vi "main.vi"() -> ()   [LabVIEW 2020]
uses:
  subvi/status/status of power_supply3.vi
  subvi/status/status of power_supply4.vi
  subvi/status/status of power_supply2.vi
  subvi/status/status of power_supply1.vi
  subvi/status/status of pump.vi
  subvi/status/status of relay.vi
  subvi/status/status of robot.vi
  subvi/status/status of worker2.vi
  subvi/status/status of worker4.vi
  subvi/status/status of worker3.vi
  subvi/status/status of worker1.vi
  subvi/status/item name.vi
  subvi/status/public_device_list.vi
  subvi/status/item name2.vi
  subvi/status/robot pause.vi
  subvi/status/stop software.vi
  subvi/status/emergency stop.vi
  subvi/status/filter_vial_No.vi
  subvi/status/skip_latter.vi
  subvi/status/skip_status.vi
  subvi/status/pause1.vi
  subvi/status/pause3.vi
  subvi/status/pause2.vi
  subvi/status/pause4.vi
  subvi/status/time1.vi
  subvi/status/time2.vi
  subvi/status/time3.vi
  subvi/status/time4.vi
  subvi/status/experiment_No.vi
  <vilib>/NI/Modbus Library/API/Wrapper/Create Serial Master.vi
  subvi/robot/subvi/Robot-HL/small_scara_interface/small_scara_interface.lvlib
  <vilib>/NI/Modbus Library/API/Wrapper/API Main.lvlib
panel:
  in  "robot pause":bool
  in  "stop software":bool
  in  "emergency stop":bool
  in  "Main interface":T1(tab)
  in  "release occupy":bool
  in  "pump load":bool
  in  "power_supply2 load":bool
  in  "motor load":bool
  in  "power_supply1 load":bool
  in  "robot load":bool
  in  "power_supply2":refnum<visa-resource-name>
  in  "power_supply":refnum<visa-resource-name>
  out "robot_busy/ready":bool
  out "pump_busy/ready":bool
  out "worker1_busy/ready":bool
  out "worker2_busy/ready":bool
  out "worker3_busy/ready":bool
  out "worker4_busy/ready":bool
  in  "start":bool
  in  "user.xls path":path=path "C:/Users/Mogroup-3/Desktop/AutoChem_test/user.xls"
  in  "Python version":string="3.11"
  out "power_supply4_busy/ready":bool
  out "power_supply1_busy/ready":bool
  out "power_supply3_busy/ready":bool
  out "power_supply2_busy/ready":bool
  out "filter_vial_No":i32
  out "relay_busy/ready":bool
  in  "pump":refnum<visa-resource-name>
  in  "motor":refnum<visa-resource-name>
  in  "filter_vial_No initial":i32
  in  "pause4":bool
  in  "pause2":bool
  in  "pause3":bool
  in  "pause1":bool
  in  "Refresh":bool
  in  "device log":i32(listbox)
  in  "experiment information":i32(listbox)
  out "start time 1":timestamp
  out "during time 1/s":dbl
  out "start time 2":timestamp
  out "during time 2/s":dbl
  out "start time 3":timestamp
  out "start time 4":timestamp
  out "during time 3/s":dbl
  out "during time 4/s":dbl
  in  "pump test":bool
  in  "channel":string
  in  "volume":dbl
  in  "rate":dbl
  in  "wait_time":dbl
  in  "robot run":bool
  in  "robot axis read":bool
  out "resulting string":string
  in  "distance":sgl
  in  "x":sgl
  in  "y":sgl
  in  "z":sgl
  in  "r":sgl
  in  "speed":sgl
  in  "rough":sgl
  in  "motor test":bool
  in  "motor ID":u8
  in  "motor commamd":string
  in  "rotate rate":u16
  in  "power_supply test":bool
  in  "Channel (1: Channel 1)":i32(ring)=1 items=["Channel 1"=1, "Channel 2"=2]
  in  "command":string
  in  "Enable Output (T: Enable)":bool=TRUE
  in  "Channel (1: Channel 1) 2":i32(ring)=1 items=["Channel 1"=1, "Channel 2"=2]
  in  "command 2":string
  in  "power_supply test 2":bool
  in  "Enable Output (T: Enable) 2":bool=TRUE
  # "Connection COM ports table"
  # "power_supply_busy/ready"
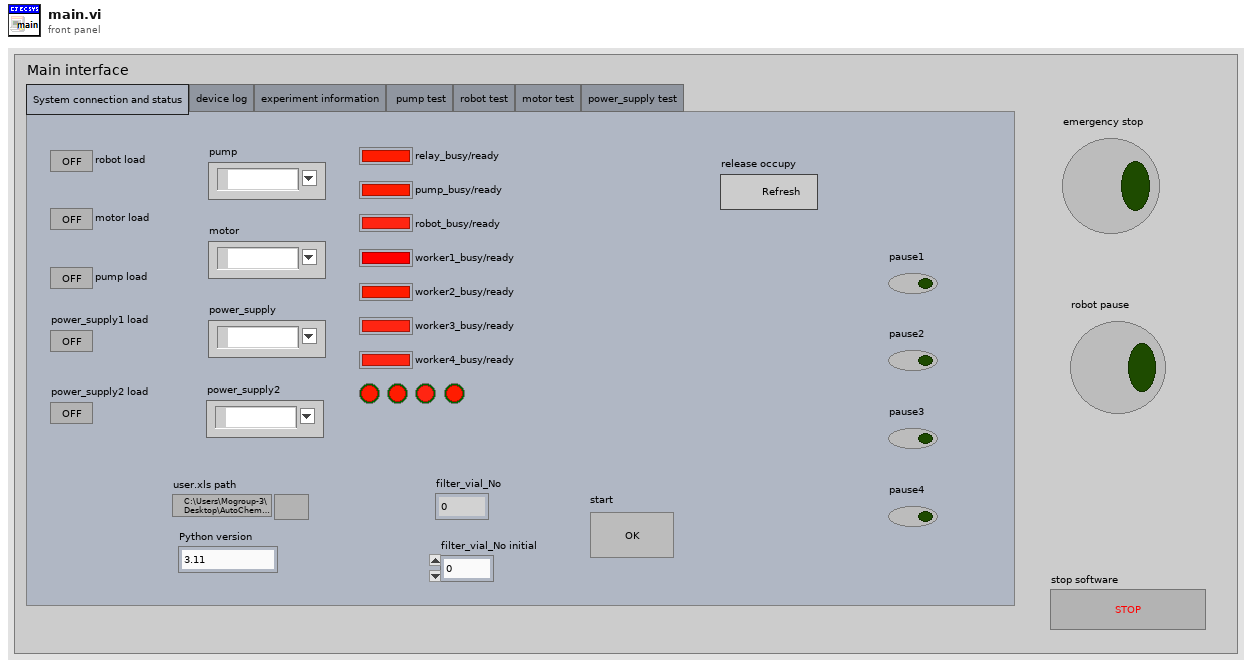
[diagram p1: front panel]
types:
  T1 = enum32{"System connection and status", "device log", "experiment information", " pump test", "robot test", "motor test", "power_supply test"}
  T2 = cluster{"start time 1":timestamp, "during time 1/s":dbl}
  T3 = cluster{"start time 2":timestamp, "during time 2/s":dbl}
  T4 = cluster{"start time 3":timestamp, "during time 3/s":dbl}
  T5 = cluster{"start time 4":timestamp, "during time 4/s":dbl}
  T6 = cluster{"x":sgl, "y":sgl, "z":sgl, "angle1":sgl, "angle2":sgl, "rotation":sgl}
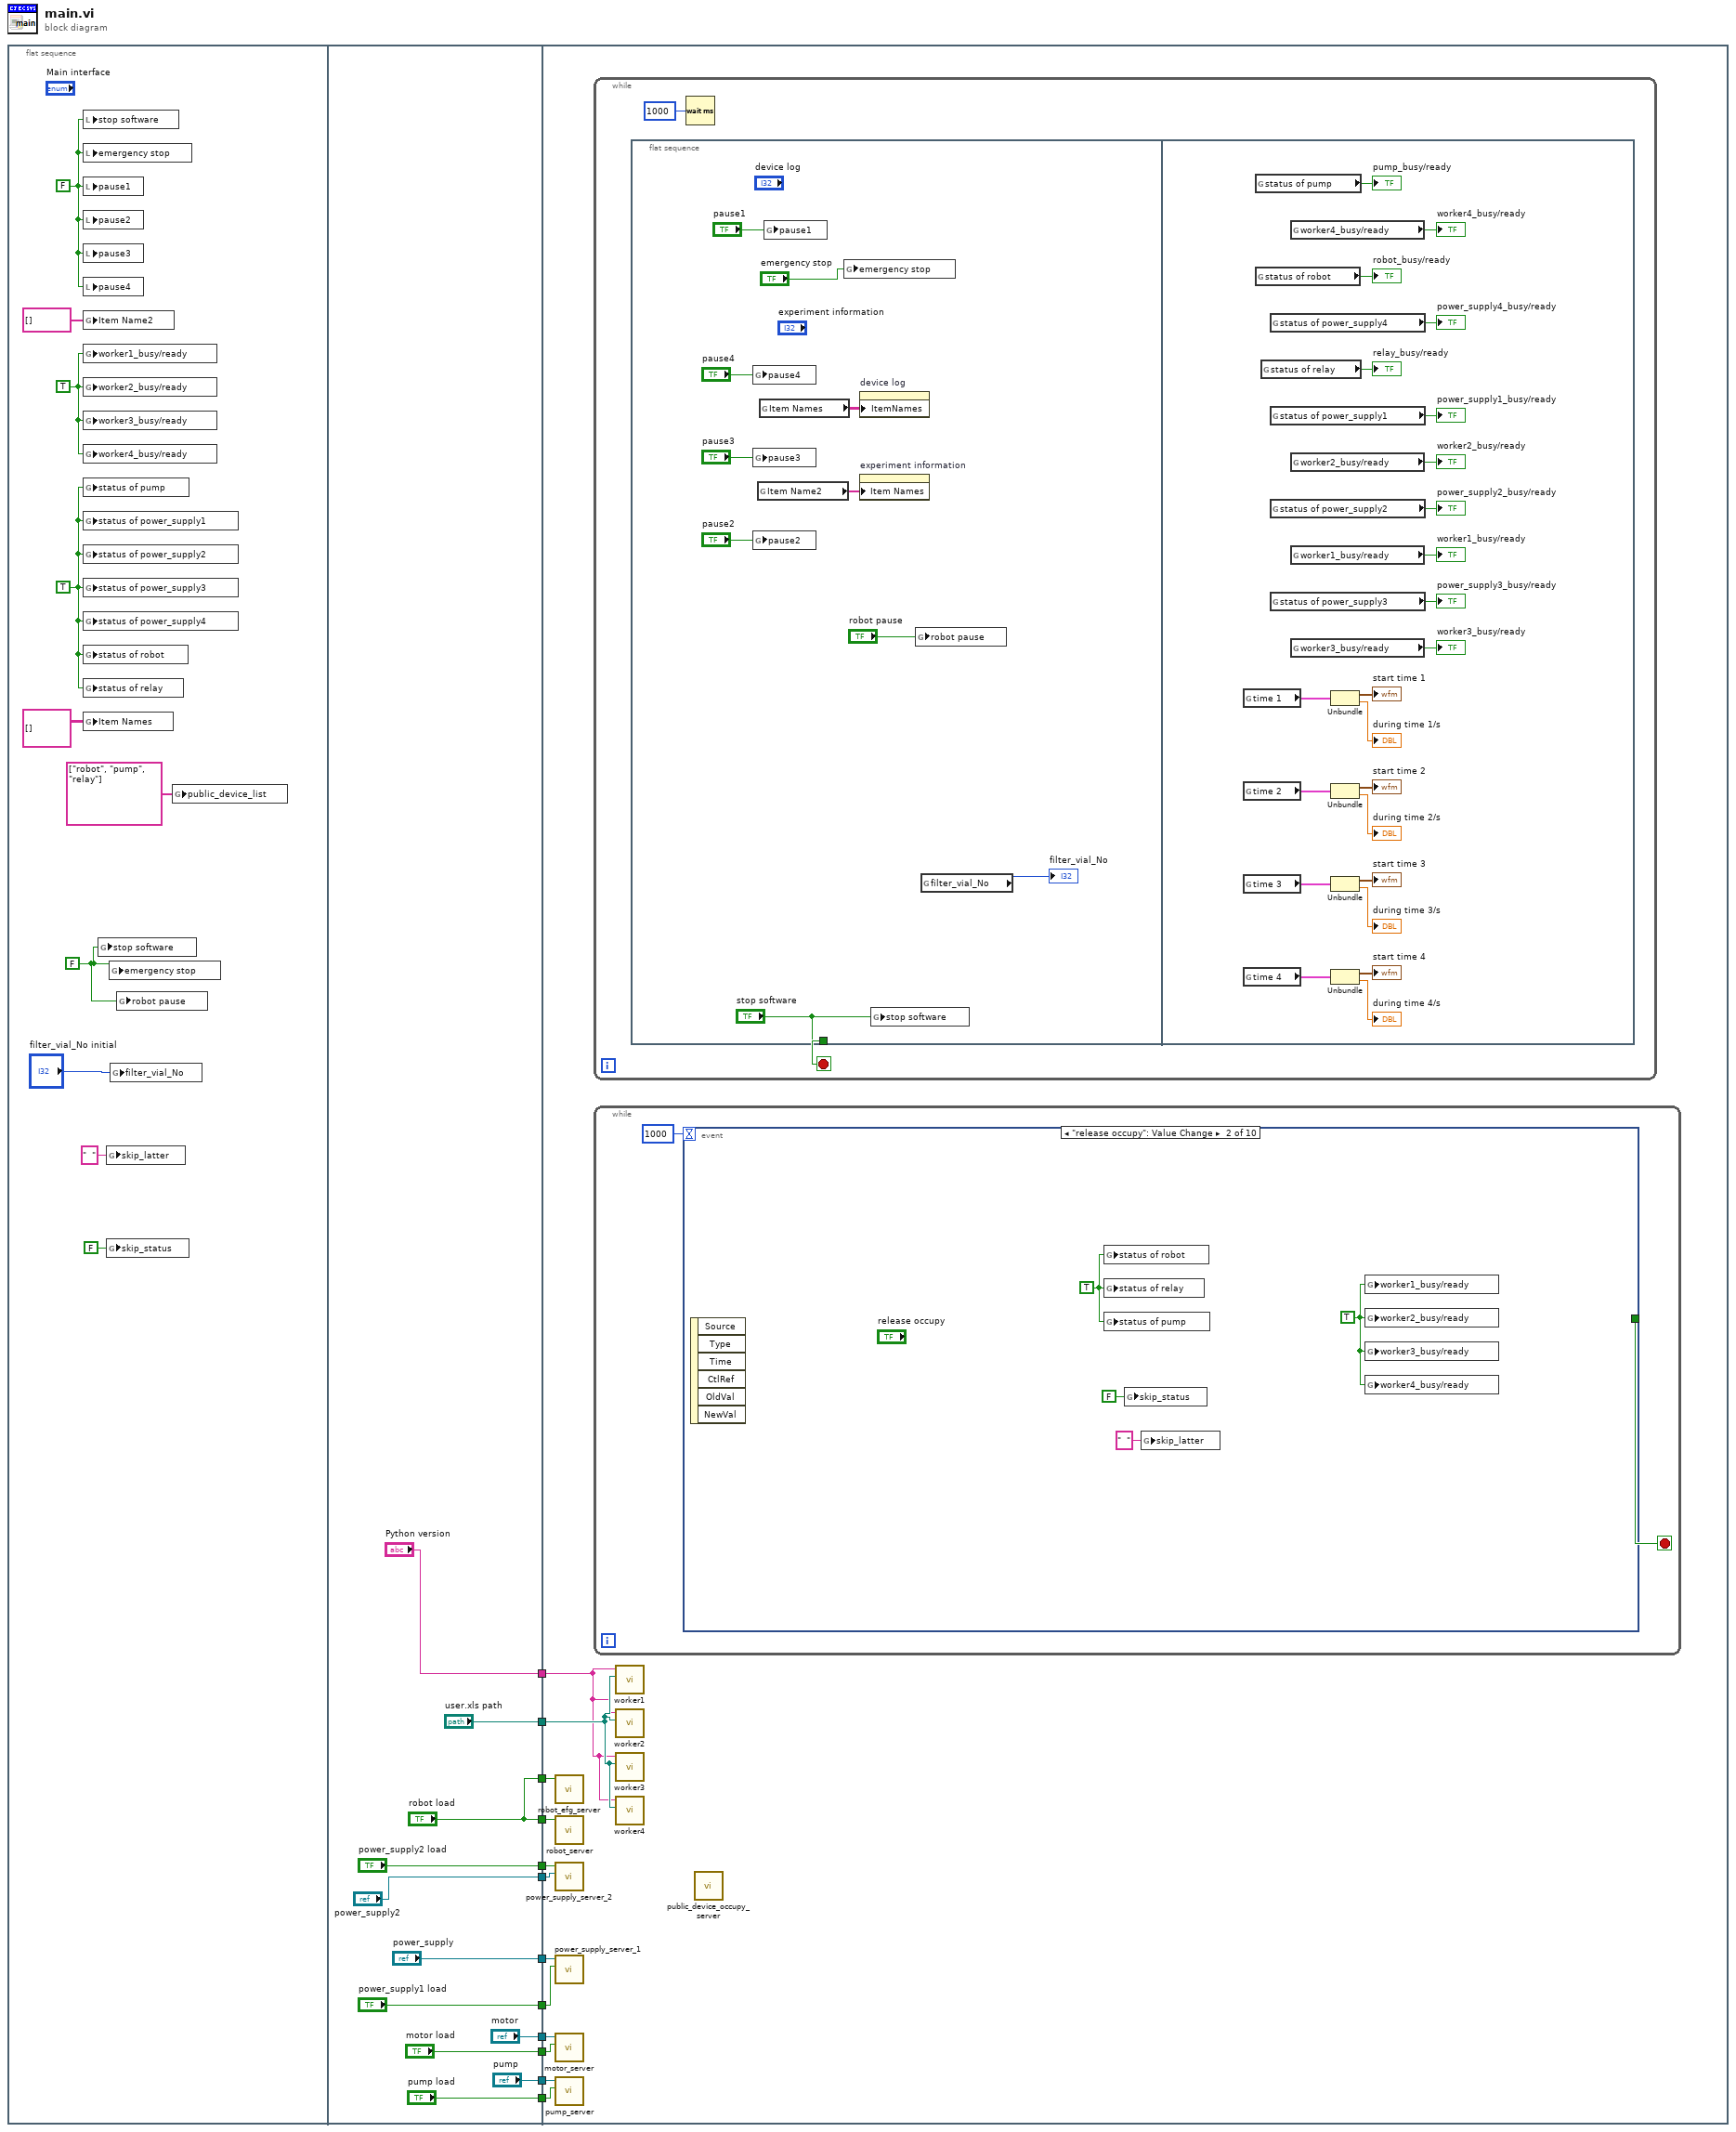
[diagram p0: block diagram]
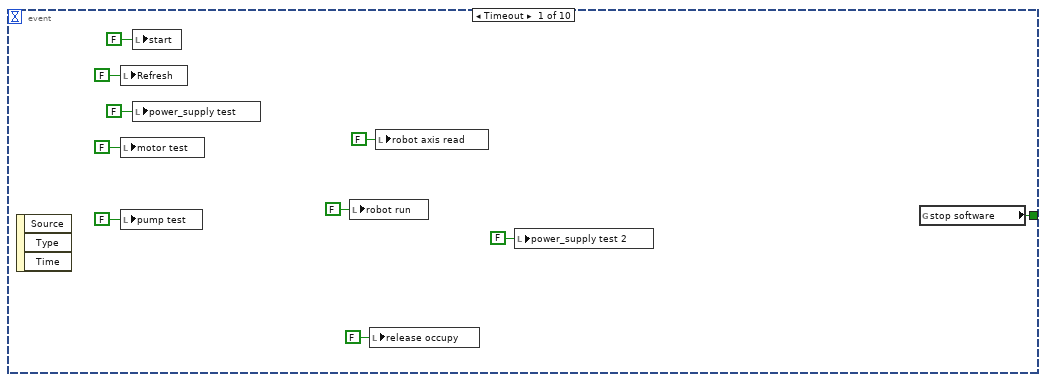
[diagram p2: hidden frame]
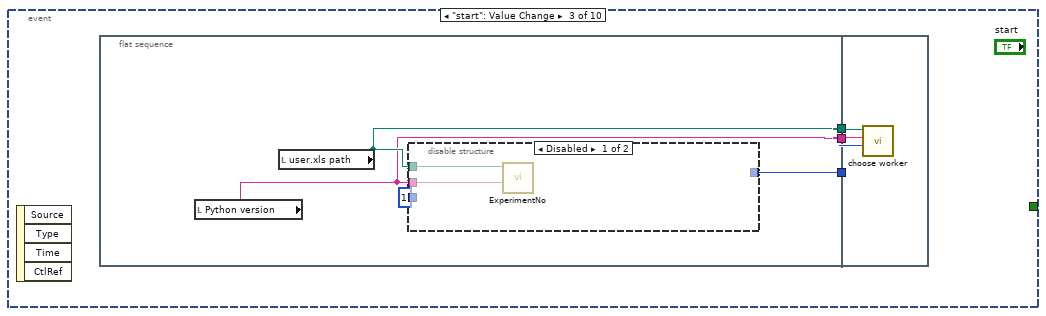
[diagram p3: hidden frame]
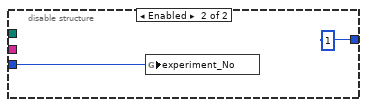
[diagram p4: hidden frame]
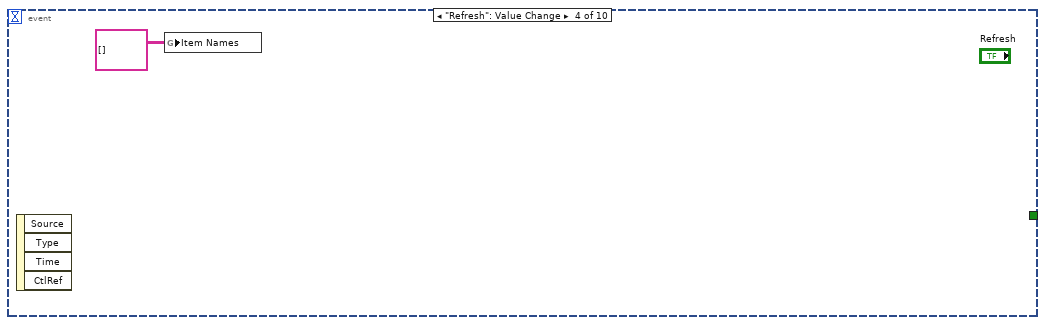
[diagram p5: hidden frame]
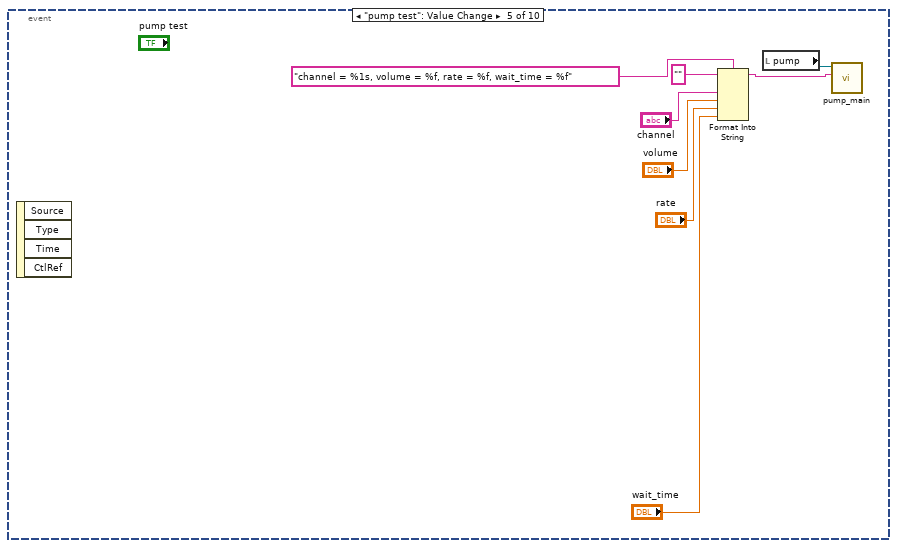
[diagram p6: hidden frame]
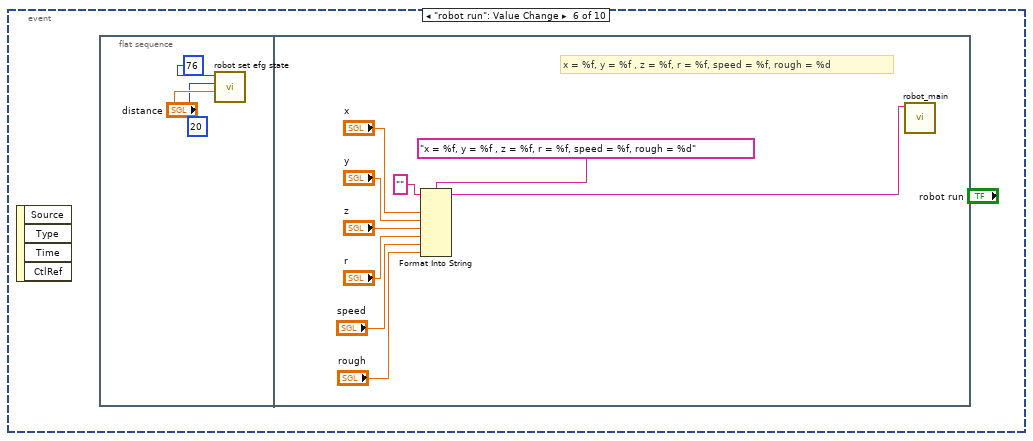
[diagram p7: hidden frame]
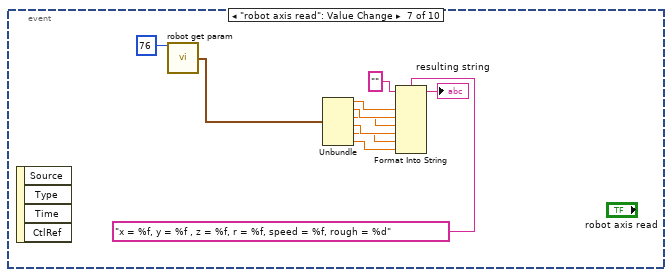
[diagram p8: hidden frame]
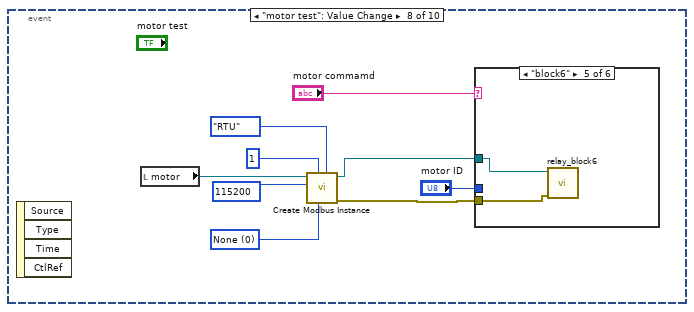
[diagram p9: hidden frame]
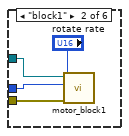
[diagram p11: hidden frame]
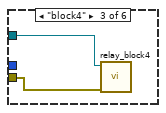
[diagram p12: hidden frame]
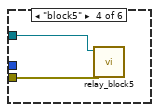
[diagram p13: hidden frame]
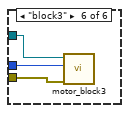
[diagram p14: hidden frame]
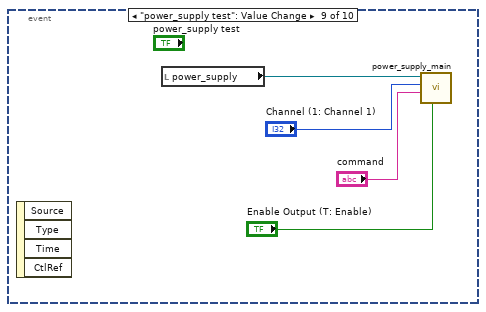
[diagram p15: hidden frame]
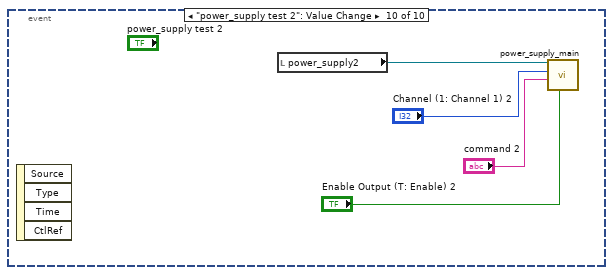
[diagram p16: hidden frame]
diagram:
  n1 = flat-sequence {
    tunnel: ["power_supply"] -> w12
    tunnel: ["motor"] -> w11
    tunnel: ["pump"] -> w10
    tunnel: ["robot load"] -> w9
    tunnel: ["power_supply1 load"] -> w8
    tunnel: ["motor load"] -> w7
    tunnel: ["pump load"] -> w6
    tunnel: ["power_supply2 load"] -> w5
    tunnel: ["power_supply2"] -> w4
    tunnel: ["user.xls path"] -> w3
    tunnel: ["Python version"] -> w2
    tunnel: ["robot load"] -> w1
    tunnel: w12 -> [w45]
    tunnel: w11 -> [w44]
    tunnel: w10 -> [w43]
    tunnel: w9 -> [w42]
    tunnel: w8 -> [w41]
    tunnel: w7 -> [w40]
    tunnel: w6 -> [w39]
    tunnel: w5 -> [w37]
    tunnel: w4 -> [w36]
    tunnel: w3 -> [w35]
    tunnel: w2 -> [w34]
    tunnel: w1 -> [w38]
    frame #0 {
      w15 = FALSE ("emergency stop")
      w21 = TRUE ("worker1_busy/ready")
      w19 = TRUE ("status of pump")
      w18 = FALSE ("stop software")
      n2 = local write "stop software"(w18) -> ()
      n3 = local write "emergency stop"(w18) -> ()
      n4 = local write "pause1"(w18) -> ()
      n5 = local write "pause2"(w18) -> ()
      n6 = local write "pause3"(w18) -> ()
      n7 = local write "pause4"(w18) -> ()
      n8 = global write "item name2.vi" "Item Name2"(string[] [] ("Item Name2")) -> ()
      n9 = global write "status of worker1.vi" "worker1_busy/ready"(w21) -> ()
      n10 = global write "status of worker2.vi" "worker2_busy/ready"(w21) -> ()
      n11 = global write "status of worker3.vi" "worker3_busy/ready"(w21) -> ()
      n12 = global write "status of worker4.vi" "worker4_busy/ready"(w21) -> ()
      n13 = global write "status of pump.vi" "status of pump"(w19) -> ()
      n14 = global write "status of power_supply1.vi" "status of power_supply1"(w19) -> ()
      n15 = global write "status of power_supply2.vi" "status of power_supply2"(w19) -> ()
      n16 = global write "status of power_supply3.vi" "status of power_supply3"(w19) -> ()
      n17 = global write "status of power_supply4.vi" "status of power_supply4"(w19) -> ()
      n18 = global write "status of robot.vi" "status of robot"(w19) -> ()
      n19 = global write "status of relay.vi" "status of relay"(w19) -> ()
      n20 = global write "item name.vi" "Item Names"(string[][] [] ("Item Names")) -> ()
      n21 = global write "stop software.vi" "stop software"(w15) -> ()
      n22 = global write "skip_latter.vi" "skip_latter"("  " ("skip_latter")) -> ()
      n23 = global write "skip_status.vi" "skip_status"(FALSE ("skip_status")) -> ()
      n24 = global write "emergency stop.vi" "emergency stop"(w15) -> ()
      n25 = global write "filter_vial_No.vi" "filter_vial_No"("filter_vial_No initial") -> ()
      n26 = global write "robot pause.vi" "robot pause"(w15) -> ()
      n27 = global write "public_device_list.vi" "public_device_list"(string[] ["robot", "pump", "relay"] ("Array")) -> ()
    }
    frame #1 {
    }
    frame #2 {
      n28 = call "robot_efg_server.vi"("efg load"=w38) -> ()  [unwired: 11 in]
      n29 = call "robot_server.vi"("robot load"=w42) -> ()  [unwired: 11 in]
      n30 = call "power_supply_server_2.vi"("power_supply 3&4"=w36, "power_supply2 load"=w37) -> ()  [unwired: 10 in]
      n31 = call "power_supply_server_1.vi"("power_supply1 load"=w41, "power_supply 1&2"=w45) -> ()  [unwired: 10 in]
      n32 = call "motor_server.vi"("motor load"=w40, "motor"=w44) -> ()  [unwired: 10 in]
      n33 = call "pump_server.vi"("pump load"=w39, "Serial Port in"=w43) -> ()  [unwired: 10 in]
      n34 = while {
        stop <- w140 stop-if-true
        n35 = flat-sequence {
          tunnel: ["stop software"] -> w140
          frame #0 {
            n36 = global write "pause4.vi" "pause4"("pause4") -> ()
            n37 = global write "pause3.vi" "pause3"("pause3") -> ()
            n38 = global write "pause2.vi" "pause2"("pause2") -> ()
            n39 = global read "item name2.vi" "Item Name2"() -> (w144:string[])
            n40 = global read "item name.vi" "Item Names"() -> (w149:string[][])
            n41 = global write "pause1.vi" "pause1"("pause1") -> ()
            n42 = global write "emergency stop.vi" "emergency stop"("emergency stop") -> ()
            n43 = property on="device log" class="MCListbox (strict)"("ItemNames"=w149) -> ()  [unwired: 2 in, 2 out]
            n44 = property on="experiment information" class="LstBox (strict)"("Item Names"=w144) -> ()  [unwired: 2 in, 2 out]
            n45 = global write "stop software.vi" "stop software"("stop software") -> ()
            n46 = global write "robot pause.vi" "robot pause"("robot pause") -> ()
            n47 = global read "filter_vial_No.vi" "filter_vial_No"() -> (→"filter_vial_No":i32)
          }
          frame #1 {
            n48 = global read "time1.vi" "time 1"() -> (w163:T2)
            n49 = global read "time2.vi" "time 2"() -> (w160:T3)
            n50 = global read "time3.vi" "time 3"() -> (w157:T4)
            n51 = global read "time4.vi" "time 4"() -> (w154:T5)
            n52 = global read "status of pump.vi" "status of pump"() -> (→"pump_busy/ready":bool)
            n53 = global read "status of robot.vi" "status of robot"() -> (→"robot_busy/ready":bool)
            n54 = global read "status of relay.vi" "status of relay"() -> (→"relay_busy/ready":bool)
            n55 = global read "status of power_supply4.vi" "status of power_supply4"() -> (→"power_supply4_busy/ready":bool)
            n56 = global read "status of power_supply1.vi" "status of power_supply1"() -> (→"power_supply1_busy/ready":bool)
            n57 = global read "status of power_supply2.vi" "status of power_supply2"() -> (→"power_supply2_busy/ready":bool)
            n58 = global read "status of power_supply3.vi" "status of power_supply3"() -> (→"power_supply3_busy/ready":bool)
            n59 = global read "status of worker4.vi" "worker4_busy/ready"() -> (→"worker4_busy/ready":bool)
            n60 = global read "status of worker2.vi" "worker2_busy/ready"() -> (→"worker2_busy/ready":bool)
            n61 = global read "status of worker1.vi" "worker1_busy/ready"() -> (→"worker1_busy/ready":bool)
            n62 = global read "status of worker3.vi" "worker3_busy/ready"() -> (→"worker3_busy/ready":bool)
            n63 = Unbundle(w163) -> ("start time 1"=→"start time 1":timestamp, "during time 1/s"=→"during time 1/s":dbl)
            n64 = Unbundle(w160) -> ("start time 2"=→"start time 2":timestamp, "during time 2/s"=→"during time 2/s":dbl)
            n65 = Unbundle(w157) -> ("start time 3"=→"start time 3":timestamp, "during time 3/s"=→"during time 3/s":dbl)
            n66 = Unbundle(w154) -> ("start time 4"=→"start time 4":timestamp, "during time 4/s"=→"during time 4/s":dbl)
          }
        }
        n67 = Wait (ms)(milliseconds to wait=u32 1000) -> ()  [unwired: 1 out]
      }
      n68 = while {
        stop <- w47 stop-if-true
        n69 = event shown="[1] \"release occupy\": Value Change" {
          selector: _ -> [_ _ _ _ _ _ _ _ _ _]
          dyn-events: _ -> [_ _ _ _ _ _ _ _ _ _]
          timeout: 1000 -> [_ _ _ _ _ _ _ _ _ _]
          tunnel: [w56 _ _ _ _ _ _ _ _ _] -> w47
          event Timeout {
            n70 = event-data() -> ()  [unwired: 1 in, 3 out]
            n71 = local write "Refresh"(FALSE ("Refresh")) -> ()
            n72 = local write "motor test"(FALSE ("motor test")) -> ()
            n73 = local write "pump test"(FALSE ("robot test")) -> ()
            n74 = local write "start"(FALSE ("OK Button")) -> ()
            n75 = local write "power_supply test"(FALSE ("power_supply test")) -> ()
            n76 = local write "robot run"(FALSE ("robot run")) -> ()
            n77 = local write "release occupy"(FALSE ("release occupy")) -> ()
            n78 = local write "robot axis read"(FALSE ("robot axis read")) -> ()
            n79 = local write "power_supply test 2"(FALSE ("power_supply test 2")) -> ()
            n80 = global read "stop software.vi" "stop software"() -> (w56:bool)
          }
          event "release occupy": Value Change {
            w60 = TRUE ("worker1_busy/ready")
            w61 = TRUE ("status of pump")
            n81 = event-data() -> ()  [unwired: 1 in, 6 out]
            n82 = global write "status of robot.vi" "status of robot"(w61) -> ()
            n83 = global write "status of relay.vi" "status of relay"(w61) -> ()
            n84 = global write "status of pump.vi" "status of pump"(w61) -> ()
            n85 = global write "skip_status.vi" "skip_status"(FALSE ("skip_status")) -> ()
            n86 = global write "skip_latter.vi" "skip_latter"("  " ("skip_latter")) -> ()
            n87 = global write "status of worker1.vi" "worker1_busy/ready"(w60) -> ()
            n88 = global write "status of worker2.vi" "worker2_busy/ready"(w60) -> ()
            n89 = global write "status of worker3.vi" "worker3_busy/ready"(w60) -> ()
            n90 = global write "status of worker4.vi" "worker4_busy/ready"(w60) -> ()
          }
          event "start": Value Change {
            n91 = event-data() -> ()  [unwired: 1 in, 4 out]
            n92 = flat-sequence {
              tunnel: [w68] -> w64
              tunnel: [w66] -> w63
              tunnel: [w65] -> w62
              tunnel: w64 -> [w77]
              tunnel: w63 -> [w76]
              tunnel: w62 -> [w75]
              frame #0 {
                n93 = local read "Python version"() -> (w65:string)
                n94 = local read "user.xls path"() -> (w66:path)
                n95 = disable-structure shown="Disabled" {
                  disable-tunnel: w66 -> [w72 _]
                  disable-tunnel: w65 -> [w71 _]
                  disable-tunnel: 1 ("Numeric") -> [_ w74]
                  disable-tunnel: [_ 1 ("total")] -> w68
                  frame Disabled {
                    n96 = call "ExperimentNo.vi"("Python version"=w71, "user.xls path"=w72) -> ("total"=w70:i32, "experiment_No"=w69:i32)  [unwired: 7 in, 1 out]
                  }
                  frame Enabled {
                    n97 = global write "experiment_No.vi" "experiment_No"(w74) -> ()
                  }
                }
              }
              frame #1 {
                n98 = call "choose worker.vi"("total"=w77, "Python version"=w75, "user.xls path"=w76) -> ()  [unwired: 9 in]
              }
            }
          }
          event "Refresh": Value Change {
            n99 = event-data() -> ()  [unwired: 1 in, 4 out]
            n100 = global write "item name.vi" "Item Names"(string[][] [] ("Item Names")) -> ()
          }
          event "pump test": Value Change {
            n101 = event-data() -> ()  [unwired: 1 in, 4 out]
            n102 = Format Into String(format string="channel = %1s, volume = %f, rate = %f, wait_time = %f", initial string="", "channel", "volume", "rate", "wait_time") -> (resulting string=w79:string)  [unwired: 1 in, 1 out]
            n103 = local read "pump"() -> (w86:refnum<visa-resource-name>)
            n104 = call "pump_main.vi"("input string"=w79, "VISA resource name"=w86) -> ()  [unwired: 8 in, 2 out]
          }
          event "robot run": Value Change {
            n105 = event-data() -> ()  [unwired: 1 in, 4 out]
            n106 = flat-sequence {
              frame #0 {
                n107 = call "robot set efg state.vi"("distance"="distance", "type"=20, "robot_id"=76) -> ()  [unwired: 8 in, 1 out]
              }
              frame #1 {
                # "x = %f, y = %f , z = %f, r = %f, speed = %f, rough = %d"
                n108 = Format Into String(format string="x = %f, y = %f , z = %f, r = %f, speed = %f, rough = %d", initial string="", "x", "y", "z", "r", "speed", "rough") -> (resulting string=w97:string)  [unwired: 1 in, 1 out]
                n109 = call "robot_main.vi"("input string"=w97) -> ()  [unwired: 9 in, 2 out]
              }
            }
          }
          event "robot axis read": Value Change {
            n110 = event-data() -> ()  [unwired: 1 in, 4 out]
            n111 = call "robot get param.vi"("robot_id"=76) -> ("输出参数簇"=w108:T6)  [unwired: 11 in, 3 out]
            n112 = Unbundle(w108) -> ("x"=w105:sgl, "y"=w104:sgl, "z"=w102:sgl, "angle1"=w101:sgl, "angle2"=w100:sgl, "rotation"=w99:sgl)
            n113 = Format Into String(format string="x = %f, y = %f , z = %f, r = %f, speed = %f, rough = %d", initial string="", w105, w104, w102, w101, w100, w99) -> (resulting string=→"resulting string":string)  [unwired: 1 in, 1 out]
          }
          event "motor test": Value Change {
            w116 = u16 0 items=["None", "Odd", "Even", "Mark", "Space"] ("parity (even)")
            n114 = event-data() -> ()  [unwired: 1 in, 4 out]
            n115 = local read "motor"() -> (w112:refnum<visa-resource-name>)
            n116 = call-poly <vilib>:"Create Modbus Instance.vi"("serial type"=enum16{"RTU", "ASCII"}."RTU", "parity (even)"=w116, "unit ID"=u8 1, "baud rate"=u32 115200, "VISA resource name"=w112) -> ("error out"=w113:errorcluster, "serial master instance"=w114:refnum<class "Modbus Master.lvclass">)  [unwired: 5 in]
            n117 = case shown="\"block6\"" "motor commamd" {
              tunnel: w114 -> [_ w122 w124 w126 w128 w131]
              tunnel: w113 -> [_ w121 w123 w125 w127 w130]
              tunnel: "motor ID" -> [_ w120 _ _ _ w129]
              frame "False", Default {
              }
              frame "block1" {
                n118 = call "motor_block1.vi"("error in"=w121, "rotate rate"="rotate rate", "unit ID"=w120, "Modbus master in"=w122) -> ()  [unwired: 6 in, 2 out]
              }
              frame "block4" {
                n119 = call "relay_block4.vi"("error in"=w123, "Modbus master in"=w124) -> ()  [unwired: 8 in, 2 out]
              }
              frame "block5" {
                n120 = call "relay_block5.vi"("error in"=w125, "Modbus master in"=w126) -> ()  [unwired: 8 in, 2 out]
              }
              frame "block6" {
                n121 = call "relay_block6.vi"("error in"=w127, "Modbus master in"=w128) -> ()  [unwired: 8 in, 2 out]
              }
              frame "block3" {
                n122 = call "motor_block3.vi"("error in"=w130, "unit ID"=w129, "Modbus master in"=w131) -> ()  [unwired: 7 in, 2 out]
              }
            }
          }
          event "power_supply test": Value Change {
            n123 = event-data() -> ()  [unwired: 1 in, 4 out]
            n124 = local read "power_supply"() -> (w135:refnum<visa-resource-name>)
            n125 = call "power_supply_main.vi"("Enable Output (T: Enable)"="Enable Output (T: Enable)", "command"="command", "channel"="Channel (1: Channel 1)", "VISA resource name"=w135) -> ()  [unwired: 6 in, 2 out]
          }
          event "power_supply test 2": Value Change {
            n126 = event-data() -> ()  [unwired: 1 in, 4 out]
            n127 = local read "power_supply2"() -> (w136:refnum<visa-resource-name>)
            n128 = call "power_supply_main.vi"("Enable Output (T: Enable)"="Enable Output (T: Enable) 2", "command"="command 2", "channel"="Channel (1: Channel 1) 2", "VISA resource name"=w136) -> ()  [unwired: 6 in, 2 out]
          }
        }
      }
      n129 = call "worker1.vi"("user.xls path"=w35, "Python version"=w34) -> ()  [unwired: 8 in, 2 out]
      n130 = call "worker2.vi"("user.xls path"=w35, "Python version"=w34) -> ()  [unwired: 8 in, 2 out]
      n131 = call "worker3.vi"("user.xls path"=w35, "Python version"=w34) -> ()  [unwired: 8 in, 2 out]
      n132 = call "worker4.vi"("user.xls path"=w35, "Python version"=w34) -> ()  [unwired: 8 in, 2 out]
      n133 = call "public_device_occupy_server.vi"() -> ()  [unwired: 12 in]
    }
  }
